vi "PH_ImageOperator.Set Energy State.vi"(0 "i ref in":refnum<vi>, 5 "error in (no error)":errorcluster) -> (14 "i ref out":refnum<vi>, 19 "error out":errorcluster)   [LabVIEW 2014, in "PH_ImageOperator.lvlib"]
doc: "This VI calculatzes the state of the energy measurement and set it (in case of a change) to own attributes and the GUI element."
uses:
  PH_ImageOperator.lvlib
  PH_Basics/PH_StatusHandler/PH_StatusHandler.Status.ctl
  PH_Basics/PH_Common/PH_Common.lvlib
  PH_Basics/PH_StatusHandler/PH_StatusHandler.lvlib
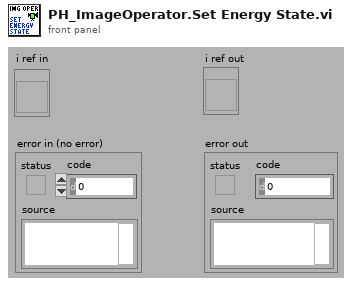
[diagram p1: front panel]
types:
  T1 = typedef "PH_StatusHandler.lvlib/PH_StatusHandler.Status.ctl" = i16
  T2 = typedef "PH_ImageOperator.lvlib/PH_ImageOperator.i attribute.ctl" = cluster{"GUI Refs":cluster{"Delete":refnum<vi>, "Calibration status":refnum<vi>, "BI subtracted":refnum<vi>, "calc Energy":refnum<vi>, "Energy: expected value":refnum<vi>, "Energy: Tolerance":refnum<vi>, "Energy calculated":refnum<vi>, "Energy":refnum<vi>, "calc Beam Anal":refnum<vi>, "Maj Diam 1/esquare":refnum<vi>, "Min Diam 1/esquare":refnum<vi>, "Azi Angle":refnum<vi>, "Min/Maj Diam esquare":refnum<vi>, "Beam analysed":refnum<vi>, "CoG - x":refnum<vi>, "CoG - y":refnum<vi>, "BA: Method":refnum<vi>, "BA: Steps":refnum<vi>, "BA: Factor":refnum<vi>, "calc Traces":refnum<vi>, "Traces: Fit Gauss":refnum<vi>, "Traces calculated":refnum<vi>, "Maj FWHM":refnum<vi>, "Min FWHM":refnum<vi>, "Major Trace":refnum<vi>, "Minor Trace":refnum<vi>, "Maj Fit Order":refnum<vi>, "Min Fit Order":refnum<vi>, "Position calculated":refnum<vi>, "Position":refnum<vi>, "Type":refnum<vi>, "Center":refnum<vi>, "exp - X":refnum<vi>, "exp - Y":refnum<vi>, "Tolerance":refnum<vi>, "f":refnum<vi>, "M":refnum<vi>, "D":refnum<vi>, "q":refnum<vi>, "Dummy Method":refnum<vi>, "Dummy Type":refnum<vi>, "Global On":refnum<vi>, "Traces: No offset":refnum<vi>, "Maj 99%":refnum<vi>, "Min 99%":refnum<vi>, "GUI FF Image":refnum<vi>, "calc Fill Factor":refnum<vi>, "FF calculated":refnum<vi>, "Fill Factor: Filter?":refnum<vi>, "FF: Damage Threshold":refnum<vi>, "FF: Threshold":refnum<vi>, "FF: max allow. Energy":refnum<vi>, "FF: Fillfactor":refnum<vi>, "Calibration data":refnum<vi>}, "List of GUIs":string[], "Calibration":cluster{"Status":T1, "Calibration data":T3, "Calibration Data File":path}, "Final Image":cluster{"BI Subtraction Failure":bool}, "Energy":cluster{"on":bool, "expected value [mJ]":dbl, "Tolerance [%]":dbl, "State":T1, "Energy [mJ]":dbl, "Unit":string, "calculated @":timestamp}, "Beam Analysis":cluster{"on":bool, "Data":T4, "Method":bool, "Steps":i32, "Factor":i32, "ROI":cluster{"Left":i32, "Top":i32, "Right":i32, "Bottom":i32}, "analysed @":timestamp}, "Trace Analysis":cluster{"on":bool, "Fit on":bool, "Maj FWHM":dbl, "Min FWHM":dbl, "Maj Fit Order":i32, "Min Fit Order":i32, "No Offset":bool, "Maj 99%":dbl, "Min 99%":dbl, "Traces":cluster{"XScaleName":string, "Y Scale Minimum":sgl, "Y Scale Maximum":sgl, "X Scale Minimum":sgl, "X Scale Maximum":sgl, "Traces":cluster{"Index":sgl[], "Trace":dbl[]}[]}[], "analysed @":timestamp}, "Position Analysis":cluster{"on":bool, "exp - X":i32, "exp - Y":i32, "focal length [mm]":dbl, "Magnification":dbl, "Delta":dbl, "Theta":dbl, "Tolerance":dbl, "Type":bool, "analysed @":timestamp}, "Fill Factor":cluster{"on":bool, "Filter on?":bool, "Threshold":dbl, "Damage Threshold [J/cm²]":dbl, "Fillfactor":dbl, "Max. allowed Energy [J]":dbl, "calculated @":timestamp}, "Statistician Service ID":i32, "Images":cluster{"Background":T5, "OP":T5, "GUI":T5, "BA: ROI":T5, "Trace: Turn":T5, "FF: Main":T5, "FF: Help":T5, "PSDB: BG":T5, "PSDB: OP":T5, "PSDB: FF":T5}}
  T3 = typedef "PH_ImageCalibrator.lvlib/PH_ImageCalibrator.Calibration Data.ctl" = cluster{"Date":string, "Time":string, "Cam Settings":cluster{"Cam ID":string, "Gain":dbl, "Brightness":dbl, "Shutter":dbl, "Cam Error":bool, "Mode":i32}, "Background Image":cluster{"Image":dbl[][], "Image Error":bool}, "Linear Calibration":cluster{"Calibration Factor":dbl, "not mm or mrad":bool}, "Energy Calibration":cluster{"Calibration Factor":dbl, "no mJ":bool}}
  T4 = typedef "PH_ImageOperator.lvlib/PH_ImageOperator.Beam Analysis Data.ctl" = cluster{"CoG-x":sgl, "CoG-y":sgl, "Maj Dim":dbl, "Min Dim":dbl, "Ellipticity":dbl, "Azimuth Angle [rad]":dbl, "Azi Angle rel to Maj?":bool}
  T5 = typedef "IMAQ Image.ctl" = refnum<image>
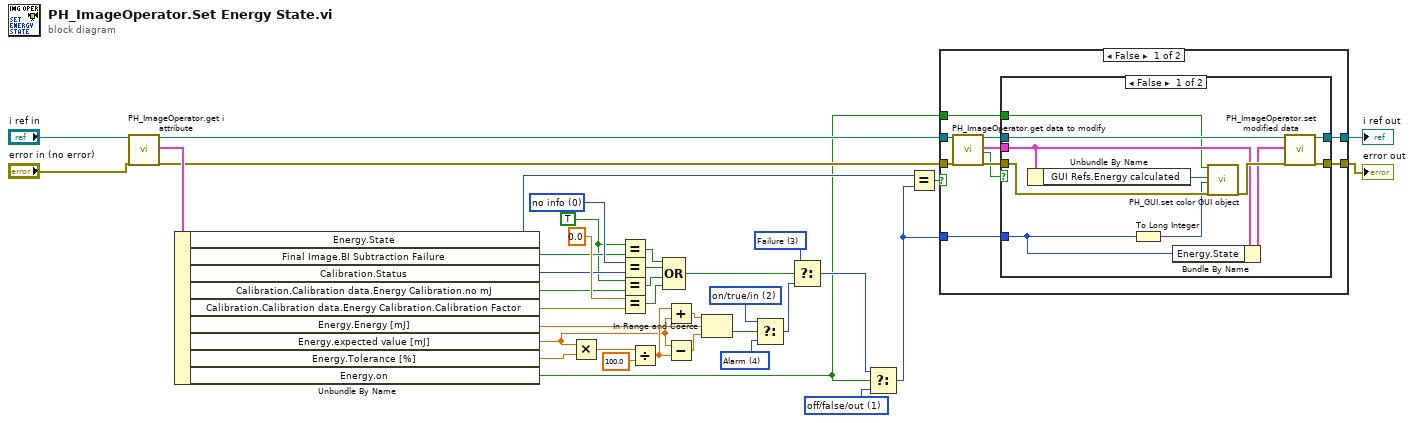
[diagram p0: block diagram]
diagram:
  w38 = T1 4 items=["no info", "off/false/out", "on/true/in", "Failure", "Alarm", "Status 1", "Status 2", "Status 3"] ("f")
  w37 = T1 2 items=["no info", "off/false/out", "on/true/in", "Failure", "Alarm", "Status 1", "Status 2", "Status 3"]
  w27 = T1 1 items=["no info", "off/false/out", "on/true/in", "Failure", "Alarm", "Status 1", "Status 2", "Status 3"] ("f")
  w26 = T1 3 items=["no info", "off/false/out", "on/true/in", "Failure", "Alarm", "Status 1", "Status 2", "Status 3"]
  w5 = TRUE ("x")
  w18 = T1 0 items=["no info", "off/false/out", "on/true/in", "Failure", "Alarm", "Status 1", "Status 2", "Status 3"] ("Calibration.Status")
  n1 = call "PH_ImageOperator.get i attribute.vi"("i ref in"="i ref in", "error in (no error)"="error in (no error)") -> ("i ref out"=w14:refnum<vi>, "i attribute"=w16:T2, "error out"=w15:errorcluster)  [unwired: 15 in]
  n2 = Unbundle By Name(w16) -> ("Energy.State"=w9:T1, "Final Image.BI Subtraction Failure"=w6:bool, "Calibration.Status"=w17:T1, "Calibration.Calibration data.Energy Calibration.no mJ"=w19:bool, "Calibration.Calibration data.Energy Calibration.Calibration Factor"=w20:dbl, "Energy.Energy [mJ]"=w3:dbl, "Energy.expected value [mJ]"=w2:dbl, "Energy.Tolerance [%]"=w29:dbl, "Energy.on"=w1:bool)
  n3 = Multiply(x=w2, y=w29) -> (x*y=w30:dbl)
  n4 = Equal?(x=w5, y=w6) -> (x = y?=w4:bool)
  n5 = Equal?(x=w18, y=w17) -> (x = y?=w22:bool)
  n6 = Equal?(x=w5, y=w19) -> (x = y?=w23:bool)
  n7 = Equal?(x=0.0, y=w20) -> (x = y?=w24:bool)
  n8 = Divide(x=w30, y=100.0) -> (x/y=w33:dbl)
  n9 = Compound Arithmetic op=OR(w4, w22, w23, w24) -> (w25:bool)
  n10 = Add(x=w33, y=w2) -> (x+y=w32:dbl)
  n11 = Subtract(x=w2, y=w33) -> (x-y=w34:dbl)
  n12 = In Range and Coerce(upper limit=w32, x=w3, lower limit=w34) -> (In Range?=w35:bool)  [unwired: 1 out]
  n13 = Select(t=w37, s=w35, f=w38) -> (s? t:f=w36:T1)
  n14 = Select(t=w26, s=w25, f=w36) -> (s? t:f=w28:T1)
  n15 = Select(t=w28, s=w1, f=w27) -> (s? t:f=w8:T1)
  n16 = Equal?(x=w9, y=w8) -> (x = y?=w7:bool)
  n17 = case shown="False" w7 {
    tunnel: w14 -> [w44 w63]
    tunnel: w15 -> [w43 w62]
    tunnel: w8 -> [w42 _]
    tunnel: [w41 w63] -> w11
    tunnel: [w40 w62] -> w10
    tunnel: w1 -> [w39 _]
    frame False {
      n18 = call "PH_ImageOperator.get data to modify.vi"("i ref in"=w44, "error in (no error)"=w43) -> ("i ref out"=w47:refnum<vi>, "i attribute"=w46:T2, "timed out"=w45:bool, "error out"=w48:errorcluster)  [unwired: 14 in]
      n19 = case shown="False" w45 {
        tunnel: w48 -> [w56 w60]
        tunnel: w47 -> [w59 w61]
        tunnel: [w58 w61] -> w41
        tunnel: [w57 w60] -> w40
        tunnel: w46 -> [w53 _]
        tunnel: w42 -> [w51 _]
        tunnel: w39 -> [w50 _]
        frame False {
          n20 = Unbundle By Name(w53) -> ("GUI Refs.Energy calculated"=w54:refnum<vi>)
          n21 = To Long Integer(number=w51) -> (32bit integer=w49:i32)
          n22 = Bundle By Name(cluster=w53, "Energy.State"=w51) -> (w52:T2)
          n23 = call "PH_GUI.set color GUI object.vi"("Visible? (true)"=w50, "GUI object Ref"=w54, "State"=w49, "error in (no error)"=w56) -> ("error out"=w55:errorcluster)  [unwired: 15 in]
          n24 = call "PH_ImageOperator.set modified data.vi"("i ref in"=w59, "i attribute"=w52, "error in (no error)"=w55) -> ("i ref out"=w58:refnum<vi>, "error out"=w57:errorcluster)  [unwired: 15 in]
        }
        frame True {
        }
      }
    }
    frame True {
    }
  }
  "i ref out" <- w11
  "error out" <- w10
